vi "manual barcode.vi"() -> ()   [LabVIEW 2015]
uses:
  Auto mode/Global 68.vi
panel:
  out "Serial no":string
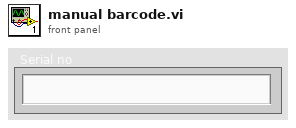
[diagram p1: front panel]
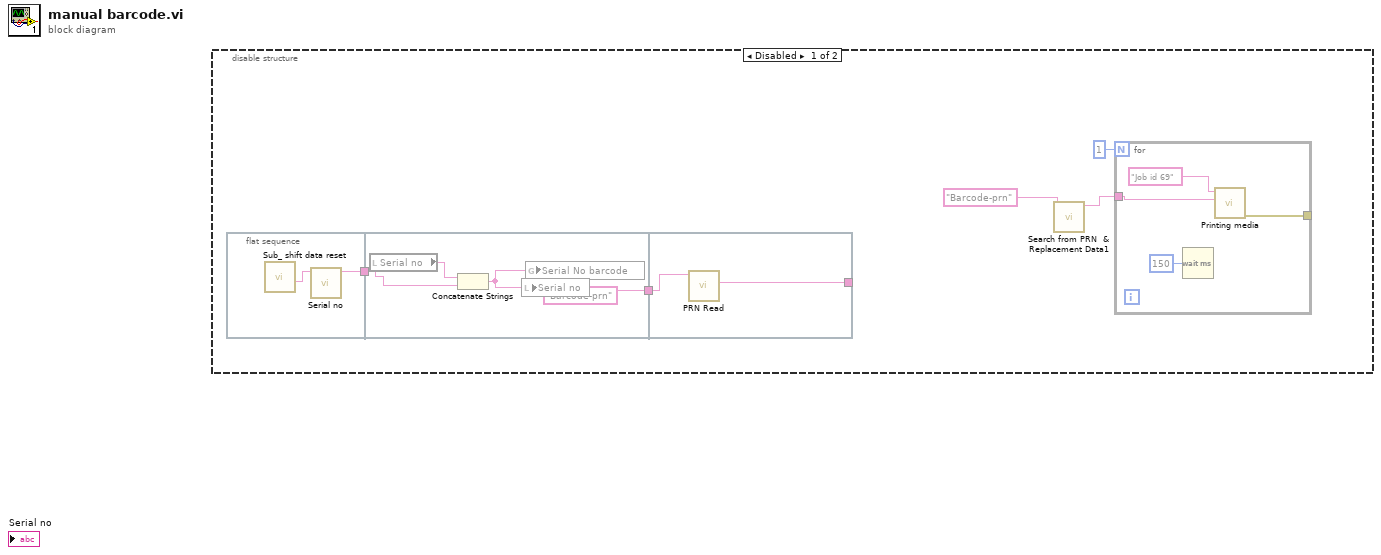
[diagram p0: block diagram]
diagram:
  n1 = disable-structure shown="Disabled" {
    frame Disabled {
      n2 = flat-sequence {
        tunnel: [w6] -> w5
        tunnel: w5 -> [w9]
        tunnel: ["Barcode-prn" ("prn")] -> w4
        tunnel: w4 -> [w13]
        tunnel: [w12] -> _
        frame #0 {
          n3 = call "Sub_ shift data reset.vi"() -> ("Serial no"=w7:string)  [unwired: 9 in, 1 out]
          n4 = call "Serial no.vi"("Serial no"=w7) -> ("String"=w6:string)  [unwired: 10 in]
        }
        frame #1 {
          n5 = local read "Serial no"() -> (w10:string)
          n6 = Concatenate Strings(w10, w9) -> (w11:string)
          n7 = local write "Serial no"(w11) -> ()
          n8 = global write "Global 68.vi" "Serial No barcode"(w11) -> ()
        }
        frame #2 {
          n9 = call "PRN Read.vi"("prn"=w13) -> ("Read Prn"=w12:string)  [unwired: 9 in, 1 out]
        }
      }
      n10 = call "Search from PRN  & Replacement Data1.vi"("PRN  Call File"="Barcode-prn" ("prn")) -> ("send on  barcode printer"=w3:string)  [unwired: 8 in, 1 out]
      n11 = for {
        N: 1 -> [_]
        tunnel: w3 -> [w17]
        tunnel: [w15] -> _
        n12 = Wait (ms)(milliseconds to wait=u32 150) -> ()  [unwired: 1 out]
        n13 = call "Printing media.vi"("send on  barcode printer"=w17, "printer name"="Job id 69") -> ("error out"=w15:errorcluster)  [unwired: 9 in]
      }
    }
    frame Enabled {
    }
  }
